vi "XML.LoadIntoCluster.vi"(6 "use cluster label as name":bool=TRUE, 7 "skip if not found?":bool, 8 "error in":errorcluster, 9 "name":string[](array[string]), 10 "clusters refs":refnum<vi>[](array[refnum]), 11 "XML file path":path=path "C:/Projects/TM-OS/trunk/Design/XML_HW_config2.xml") -> (0 "error out":errorcluster)   [LabVIEW 2019, in "Tools.lvlib"]
uses:
  Tools.lvlib
  <vilib>/xml/Load XML File.vi
  <vilib>/xml/Close Reference(Node).vi
  <vilib>/xml/NI_XML.lvlib
  <resource>/objmgr/DOMUserDefRef.rc
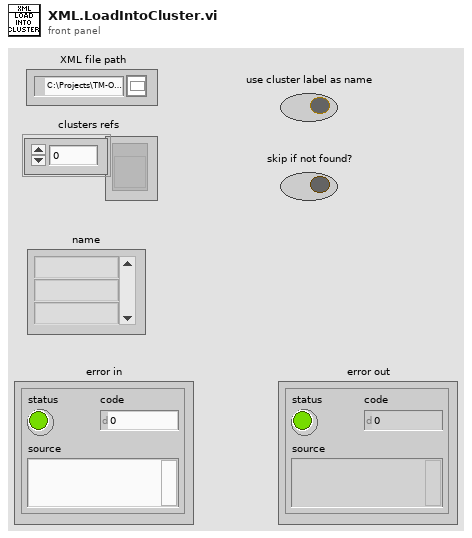
[diagram p1: front panel]
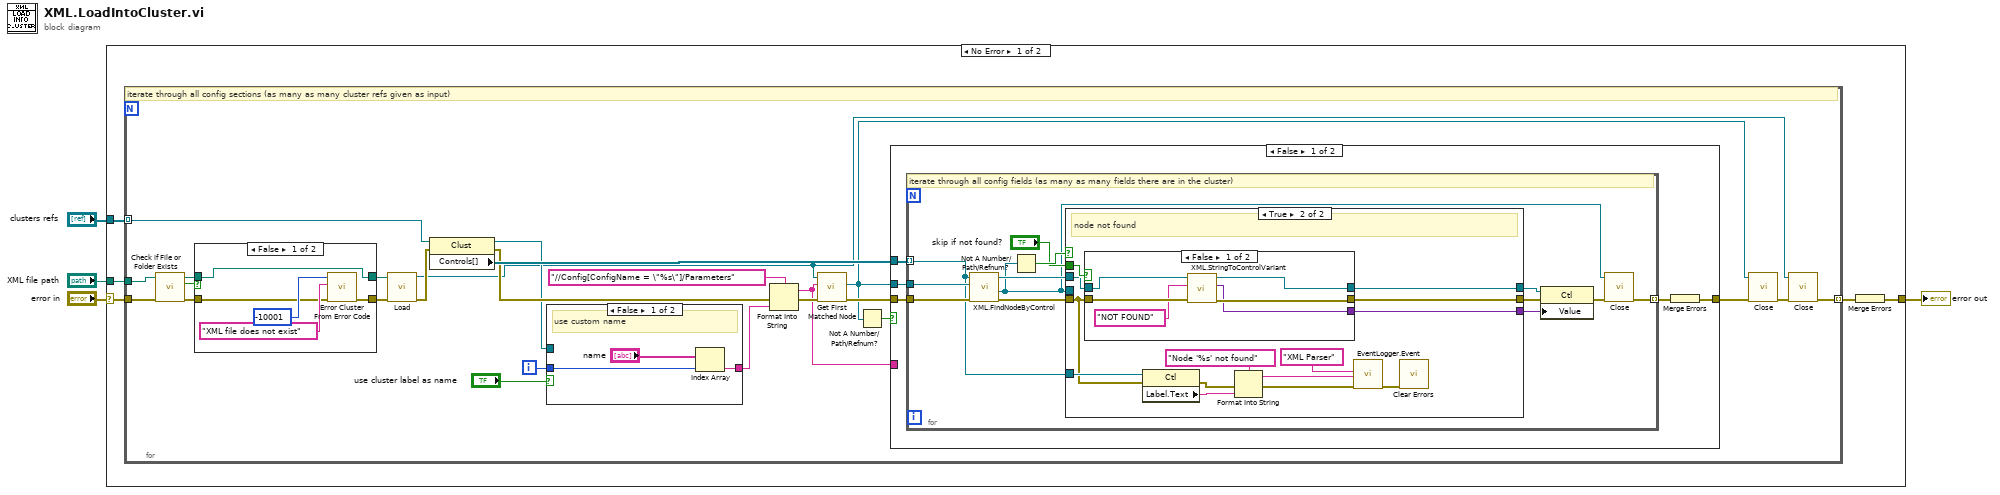
[diagram p0: block diagram]
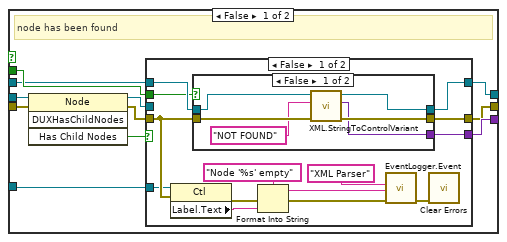
[diagram p2: hidden frame]
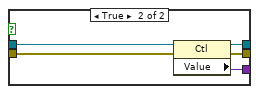
[diagram p3: hidden frame]
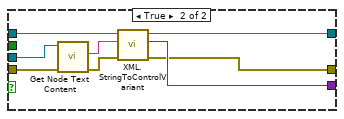
[diagram p4: hidden frame]
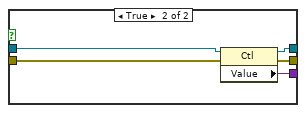
[diagram p5: hidden frame]
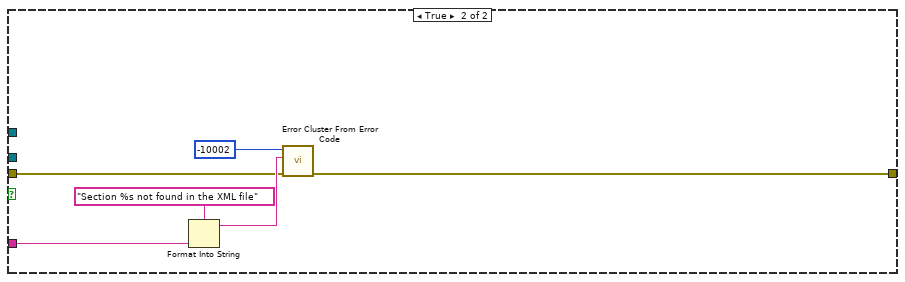
[diagram p6: hidden frame]
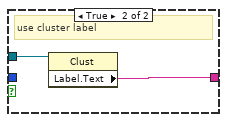
[diagram p8: hidden frame]
diagram:
  n1 = case shown="No Error" "error in" {
    selector: "error in" -> [w7 w140]
    tunnel: "clusters refs" -> [w9 _]
    tunnel: [w5 w140] -> w4
    tunnel: "XML file path" -> [w8 _]
    frame No Error {
      n2 = for {
        tunnel: w9 -> [w29] mode=indexing
        tunnel: w8 -> [w31]
        tunnel: w7 -> [w19]
        tunnel: [w22] -> w6 mode=indexing
        i -> [w25]
        # "iterate through all config sections (as many as many cluster refs given as input)"
        n3 = call <vilib>:"Check if File or Folder Exists.vi"("error in (no error)"=w19, "path"=w31) -> ("error out"=w14:errorcluster, "file or folder exists?"=w15:bool, "dup path"=w17:path)  [unwired: 7 in]
        n4 = case shown="False" w15 {
          tunnel: [w132 w133] -> w18
          tunnel: w17 -> [w129 w134]
          tunnel: [w129 w134] -> w16
          tunnel: w14 -> [w128 w133]
          frame False {
            n5 = call <vilib>:"Error Cluster From Error Code.vi"("error in (no error)"=w128, "error message (\"\")"="XML file does not exist" ("error message (\"\")"), "error code (0)"=-10001) -> ("error out"=w132:errorcluster)  [unwired: 6 in]
          }
          frame True {
          }
        }
        n6 = call-poly <vilib>:"Load.vi"("path to XML document"=w16, "error in (no error)"=w18) -> ("DOM document out"=w23:refnum<k20>, "error out"=w27:errorcluster)  [unwired: 11 in, 1 out]
        n7 = property class="Clust"(reference=w29, error in=w27) -> (reference out=w24:refnum<vi>, error out=w26:errorcluster, "Controls[]"=w34:refnum<vi>[])
        n8 = case shown="False" "use cluster label as name" {
          tunnel: [w136 w139] -> w30
          tunnel: w24 -> [_ w138]
          tunnel: w25 -> [w135 _]
          frame False {
            # "use custom name"
            n9 = Index Array(array="name", index=w135) -> (element=w136:string)
          }
          frame True {
            # "use cluster label"
            n10 = property class="Clust"(reference=w138) -> ("Label.Text"=w139:string)  [unwired: 1 in, 2 out]
          }
        }
        n11 = Format Into String(format string="//Config[ConfigName = \"%s\"]/Parameters" ("XPath expression"), error in=w26, w30) -> (resulting string=w13:string, error out=w32:errorcluster)  [unwired: 1 in]
        n12 = call <vilib>:"Get First Matched Node.vi"("error in (no error)"=w32, "XPath expression"=w13, "node in"=w23) -> ("error out"=w12:errorcluster, "node result"=w11:refnum<k20>)  [unwired: 6 in, 1 out]
        n13 = Not A Number/Path/Refnum?(number/path/refnum=w11) -> (NaN/Path/Refnum?=w10:bool)
        n14 = case shown="False" w10 {
          tunnel: w34 -> [w39 _]
          tunnel: [w35 w126] -> w21
          tunnel: w11 -> [w37 _]
          tunnel: w13 -> [_ w125]
          tunnel: w12 -> [w36 w122]
          frame False {
            n15 = for {
              tunnel: w37 -> [w52]
              tunnel: w39 -> [w40] mode=indexing
              tunnel: w36 -> [w50]
              tunnel: [w42] -> w38 mode=indexing
              # "iterate through all config fields (as many as many fields there are in the cluster)"
              n16 = call "XML.FindNodeByControl.vi"("error in (no error)"=w50, "node in"=w52, "Control in"=w40) -> ("error out"=w48:errorcluster, "found node"=w41:refnum<k20>, "Control out"=w44:refnum<vi>)  [unwired: 5 in, 1 out]
              n17 = Not A Number/Path/Refnum?(number/path/refnum=w41) -> (NaN/Path/Refnum?=w46:bool)
              n18 = case shown="True" w46 {
                tunnel: [w63 w108] -> w51
                tunnel: [w62 w110] -> w49
                tunnel: w41 -> [w61 _]
                tunnel: w48 -> [w60 w98]
                tunnel: w44 -> [w55 w107]
                tunnel: [w54 w106] -> w47
                tunnel: "skip if not found?" -> [w56 w109]
                tunnel: w40 -> [w53 w103]
                frame False {
                  # "node has been found"
                  n19 = invoke class="Node" method="DUXHasChildNodes"(reference=w61, error in=w60) -> (reference out=w58:refnum<k20>, error out=w59:errorcluster, "Has Child Nodes"=w57:bool)  [unwired: 2 in, 1 out]
                  n20 = case shown="False" w57 {
                    tunnel: [w76 w95] -> w63
                    tunnel: [w77 w91] -> w62
                    tunnel: w55 -> [w75 w90]
                    tunnel: w59 -> [w66 w94]
                    tunnel: w58 -> [_ w93]
                    tunnel: w56 -> [w74 _]
                    tunnel: [w73 w92] -> w54
                    tunnel: w53 -> [w65 _]
                    frame False {
                      n21 = property class="Ctl"(reference=w65, error in=w66) -> (error out=w68:errorcluster, "Label.Text"=w64:string)  [unwired: 1 out]
                      n22 = case shown="False" w74 {
                        tunnel: w66 -> [w81 w84]
                        tunnel: [w80 w88] -> w77
                        tunnel: [w78 w87] -> w76
                        tunnel: w75 -> [w83 w86]
                        tunnel: [w82 w85] -> w73
                        frame False {
                          n23 = call "XML.StringToControlVariant.vi"("error in (no error)"=w81, "node text"="NOT FOUND", "Control in"=w83) -> ("error out"=w80:errorcluster, "Variant"=w78:variant, "Control out"=w82:refnum<vi>)  [unwired: 6 in]
                        }
                        frame True {
                          n24 = property class="Ctl"(reference=w86, error in=w84) -> (reference out=w85:refnum<vi>, error out=w88:errorcluster, "Value"=w87:variant)
                        }
                      }
                      n25 = Format Into String(format string="Node '%s' empty", error in=w68, w64) -> (resulting string=w69:string, error out=w67:errorcluster)  [unwired: 1 in]
                      n26 = call "EventLogger.Event.vi"("error in"=w67, "Event Description"=w69, "Event Name"="XML Parser") -> ("error out"=w72:errorcluster)  [unwired: 8 in]
                      n27 = call <vilib>:"Clear Errors.vi"("error in (no error)"=w72) -> ()  [unwired: 5 in, 2 out]
                    }
                    frame True {
                      n28 = call <vilib>:"Get Node Text Content.vi"("error in (no error)"=w94, "node in"=w93) -> ("error out"=w89:errorcluster, "node text"=w96:string)  [unwired: 7 in, 1 out]
                      n29 = call "XML.StringToControlVariant.vi"("error in (no error)"=w89, "node text"=w96, "Control in"=w90) -> ("error out"=w91:errorcluster, "Variant"=w95:variant, "Control out"=w92:refnum<vi>)  [unwired: 6 in]
                    }
                  }
                }
                frame True {
                  # "node not found"
                  n30 = case shown="False" w109 {
                    tunnel: w98 -> [w116 w118]
                    tunnel: [w115 w121] -> w110
                    tunnel: [w111 w120] -> w108
                    tunnel: w107 -> [w114 w119]
                    tunnel: [w113 w117] -> w106
                    frame False {
                      n31 = call "XML.StringToControlVariant.vi"("error in (no error)"=w116, "node text"="NOT FOUND", "Control in"=w114) -> ("error out"=w115:errorcluster, "Variant"=w111:variant, "Control out"=w113:refnum<vi>)  [unwired: 6 in]
                    }
                    frame True {
                      n32 = property class="Ctl"(reference=w119, error in=w118) -> (reference out=w117:refnum<vi>, error out=w121:errorcluster, "Value"=w120:variant)
                    }
                  }
                  n33 = property class="Ctl"(reference=w103, error in=w98) -> (error out=w99:errorcluster, "Label.Text"=w102:string)  [unwired: 1 out]
                  n34 = Format Into String(format string="Node '%s' not found", error in=w99, w102) -> (resulting string=w100:string, error out=w97:errorcluster)  [unwired: 1 in]
                  n35 = call "EventLogger.Event.vi"("error in"=w97, "Event Description"=w100, "Event Name"="XML Parser") -> ("error out"=w105:errorcluster)  [unwired: 8 in]
                  n36 = call <vilib>:"Clear Errors.vi"("error in (no error)"=w105) -> ()  [unwired: 5 in, 2 out]
                }
              }
              n37 = property class="Ctl"(reference=w47, error in=w49, "Value"=w51) -> (error out=w43:errorcluster)  [unwired: 1 out]
              n38 = call-poly <vilib>:"Close.vi"("error in (no error)"=w43, "node"=w41) -> ("error out"=w42:errorcluster)  [unwired: 7 in]
            }
            n39 = Merge Errors(w38) -> (w35:errorcluster)
          }
          frame True {
            n40 = Format Into String(format string="Section %s not found in the XML file", w125) -> (resulting string=w123:string)  [unwired: 2 in, 1 out]
            n41 = call <vilib>:"Error Cluster From Error Code.vi"("error in (no error)"=w122, "error message (\"\")"=w123, "error code (0)"=-10002) -> ("error out"=w126:errorcluster)  [unwired: 6 in]
          }
        }
        n42 = call-poly <vilib>:"Close.vi"("error in (no error)"=w21, "node"=w11) -> ("error out"=w20:errorcluster)  [unwired: 7 in]
        n43 = call-poly <vilib>:"Close.vi"("error in (no error)"=w20, "node"=w23) -> ("error out"=w22:errorcluster)  [unwired: 7 in]
      }
      n44 = Merge Errors(w6) -> (w5:errorcluster)
    }
    frame Error {
    }
  }
  "error out" <- w4
